vi "ATF-Pump-CDT setter.vi"(8 "error in":errorcluster, 9 "Time Stamp":timestamp, 11 "Enum":enum16{"Write", "Read"}(ring)=enum."Read") -> (0 "error out":errorcluster, 1 "Time StampOut":timestamp)   [LabVIEW 2022 SP3]
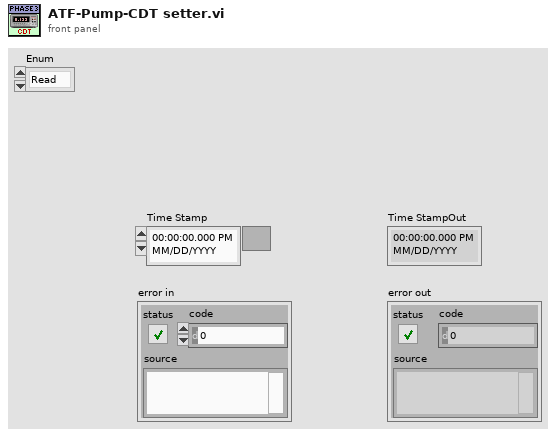
[diagram p1: front panel]
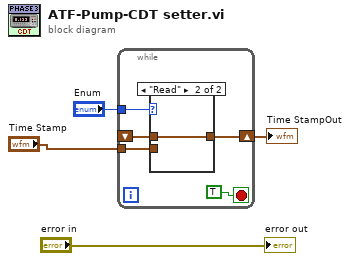
[diagram p0: block diagram]
diagram:
  n1 = while {
    tunnel: "Enum" -> [w9]
    tunnel: "Time Stamp" -> [w7]
    shift-right: [w6] -> w1
    shift-left: _ -> [w5]
    stop <- TRUE stop-if-true
    n2 = case shown="\"Read\"" w9 {
      tunnel: w7 -> [w10 _]
      tunnel: [w10 w11] -> w6
      tunnel: w5 -> [_ w11]
      frame "Write", Default {
      }
      frame "Read" {
      }
    }
  }
  "Time StampOut" <- w1
  "error out" <- "error in"
